vi "3-3.vi"() -> ()   [LabVIEW 2015]
panel:
  out "cluster 2":T1
  out "cluster":T1
  in  "Array of Strings":string[](array[string])
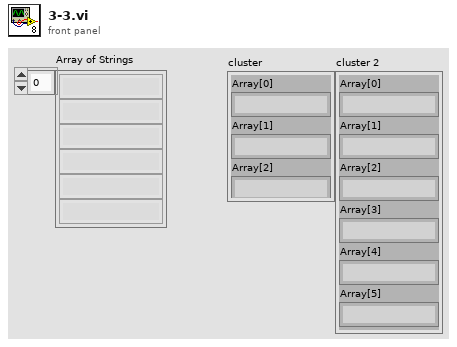
[diagram p1: front panel]
types:
  T1 = cluster{"Array[0]":string, "Array[1]":string, "Array[2]":string, "Array[3]":string, "Array[4]":string, "Array[5]":string, "Array[6]":string, "Array[7]":string, "Array[8]":string}
  T2 = cluster{"Array of Strings[0]":string, "Array of Strings[1]":string, "Array of Strings[2]":string, "Array of Strings[3]":string, "Array of Strings[4]":string, "Array of Strings[5]":string, "Array of Strings[6]":string, "Array of Strings[7]":string, "Array of Strings[8]":string}
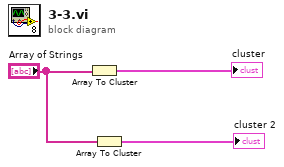
[diagram p0: block diagram]
diagram:
  n1 = Array To Cluster(array="Array of Strings") -> (cluster=→"cluster":T2)
  n2 = Array To Cluster(array="Array of Strings") -> (cluster=→"cluster 2":T2)
